vi "LV_61_Write Characters To File.vi"(0 "convert eol? (no:F)":bool, 3 "append to file? (new file:F)":bool, 4 "character string":string, 5 "file path (dialog if empty)":path) -> (2 "new file path (Not A Path if cancelled)":path)   [LabVIEW 2016]
doc: "Writes a <B>character string</B> to a new byte stream file or appends the string to an existing file. The VI opens or creates the file before writing to it and closes it afterwards."
panel:
  in  "prompt":string="Choose file to write."
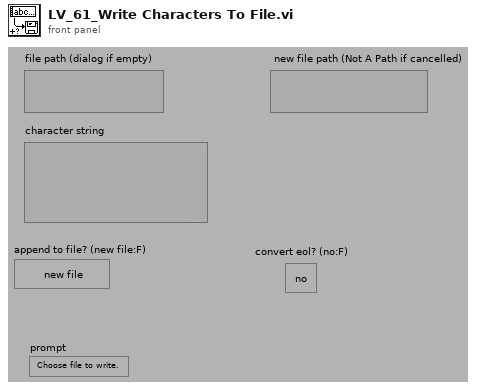
[diagram p1: front panel]
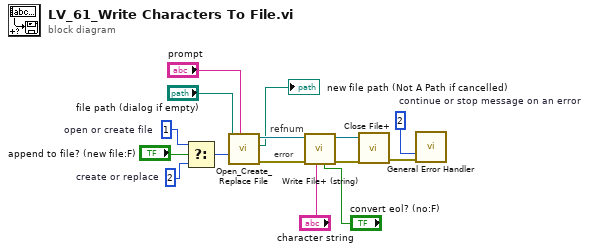
[diagram p0: block diagram]
diagram:
  w5 = i16 2  # create or replace
  w13 = 2  # continue or stop message on an error
  w8 = i16 1  # open or create file
  # "error"
  # "refnum"
  n1 = Select(t=w8, s="append to file? (new file:F)", f=w5) -> (s? t:f=w10:i16)
  n2 = call <vilib>:"Open_Create_Replace File.vi"("prompt"="prompt", "function (open:0)"=w10, "file path"="file path (dialog if empty)") -> ("error out"=w14:errorcluster, "new file path"=→"new file path (Not A Path if cancelled)":path, "refnum"=w4:refnum<file>)  [unwired: 5 in, 1 out]
  n3 = call <vilib>:"Write File+ (string).vi"("convert eol? (no:F)"="convert eol? (no:F)", "string"="character string", "error in (no error)"=w14, "refnum"=w4) -> ("error out"=w12:errorcluster, "dup refnum"=w11:refnum<file>)  [unwired: 3 in, 1 out]
  n4 = call <vilib>:"Close File+.vi"("error in (no error)"=w12, "refnum"=w11) -> ("error out"=w9:errorcluster)  [unwired: 3 in, 2 out]
  n5 = call <vilib>:"General Error Handler.vi"("type of dialog (OK msg:1)"=w13, "error in (no error)"=w9) -> ()  [unwired: 9 in, 5 out]
